vi "Main.vi"() -> ()   [LabVIEW 2023]
panel:
  in  "User interface":T1(tab)
  in  "User entries":enum32{""}(tab)
  in  "Customization":enum32{"Customization"}(tab)
  in  "Marker shape":string
  in  "Marker size":i32
  in  "PNG file path":path=path "/Users/leogallacio/Downloads/N8.png"
  in  "Colors":enum32{"Colors"}(tab)
  out "Corners":u32(colorbox)
  out "Traces":u32[](array[colorbox])
  in  "Size":enum32{"Size"}(tab)
  out "Depth":i32
  out "Width":i16
  out "Height":i16
  out "stdout":string
  out "PNG picture":picture
  out "Traces.txt":string
  out "Script.m":string
  in  "Loop FOR 1":enum32{"Loop FOR 1"}(tab)
  in  "Arrays":enum32{"Arrays"}(tab)
  out "Pixels colors (uchar)":u32[](array[numeric])
  out "Pixels colors (CLUT)":u8[](array[numeric])
  out "Corners color (CLUT)":i32
  out "Traces colors (RGB)":u8[][](array[numeric])
  out "Traces colors (CLUT)":i32[](array[numeric])
  out "Traces colors string (RGB)":string[](array[string])
  in  "Script.m":enum32{"Script.m"}(tab)
  in  "Extract.c output string scan":enum32{"Extract.c output string scan"}(tab)
  in  "T: tt1 tt2 tt3 ...":enum32{"T: tt1 tt2 tt3 ..."}(tab)
  in  "C: cc":enum32{"C: cc"}(tab)
  in  "Loop FOR 2":enum32{"Loop FOR 2"}(tab)
  out "Number of Traces":i32
  in  "LabVIEW":enum32{"LabVIEW"}(tab)
  out "VI folder":path
  out "PNG file name":string
  in  "MATLAB":enum32{"MATLAB"}(tab)
  out "Extract path":path
  out "Script.m path":path
  out "PDF file path":path
  in  "C":enum32{"C"}(tab)
  out "Pixmap.bin path":path
  out "Traces.txt path":path
  in  "MATLAB":enum32{"MATLAB"}(tab)
  out "CallMATLAB out":errorcluster
  out "CallMATLAB error":string
  in  "C":enum32{"C"}(tab)
  out "Extract.c error":string
  out "error out":errorcluster
  out "Pixmap.bin error out":errorcluster
  out "Extract error":errorcluster
  out "TracesRead error":errorcluster
  out "ScriptWrite error out":errorcluster
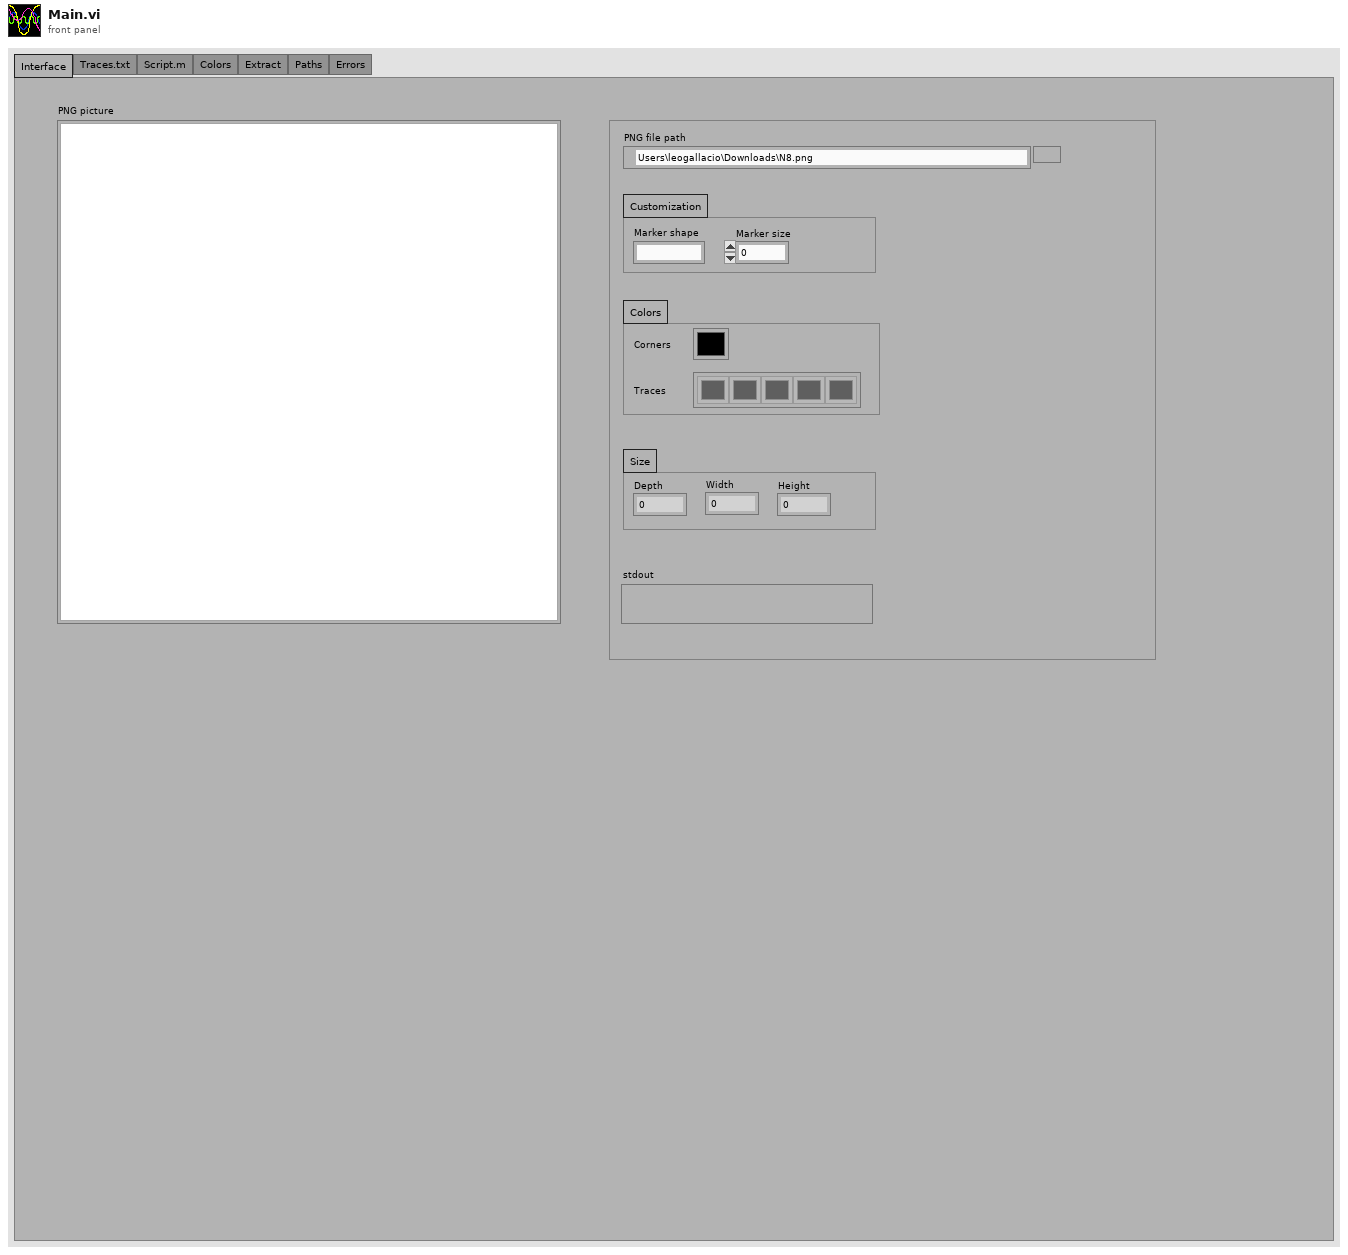
[diagram p1: front panel]
types:
  T1 = enum32{"Interface", "Traces.txt", "Script.m", "Colors", "Extract", "Paths", "Errors"}
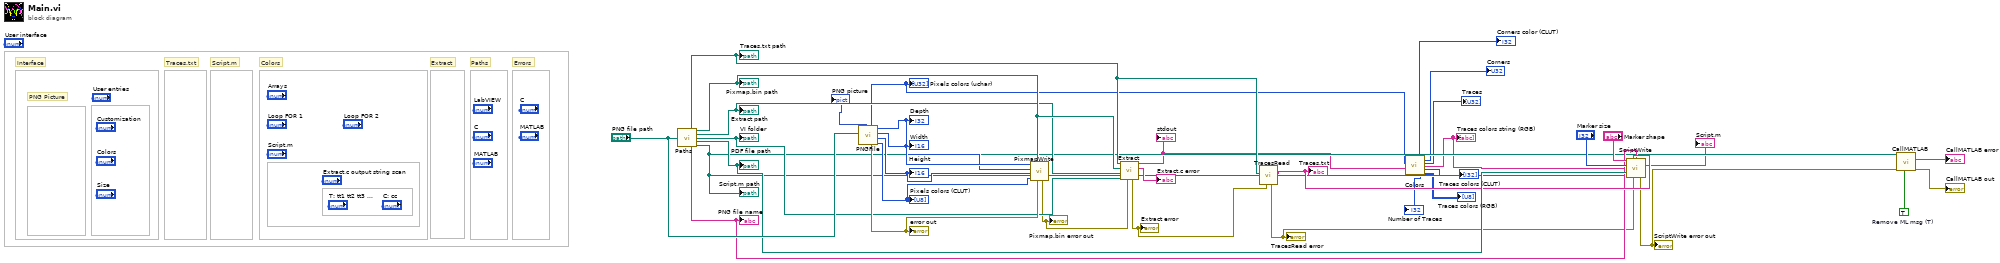
[diagram p0: block diagram]
diagram:
  w33 = TRUE  # Remove ML msg (T)
  # "PNG Picture"
  # "Errors"
  # "Paths"
  # "Extract"
  # "Colors"
  # "Script.m"
  # "Traces.txt"
  # "Interface"
  n1 = call "Paths.vi"("PNG file path"="PNG file path") -> ("Traces.txt path"=w21:path, "Pixmap.bin path"=w26:path, "Extract path"=w25:path, "VI folder"=w24:path, "PDF file path"=w17:path, "PNG file name"=w15:string, "Script.m path"=w13:path)  [unwired: 8 in]
  "Traces.txt path" <- w21
  "Pixmap.bin path" <- w26
  "Extract path" <- w25
  "VI folder" <- w24
  "PDF file path" <- w17
  "Script.m path" <- w13
  "PNG file name" <- w15
  n2 = call "PNGFile.vi"("PNG file path"="PNG file path") -> ("Pixels colors (CLUT)"=w28:u8[], "Height"=w29:i16, "Width"=w30:i16, "Depth"=w31:i32, "PNGFile error"=w27:errorcluster, "Pixels colors (uchar)"=w12:u32[], "PNG picture"=→"PNG picture":picture)  [unwired: 4 in]
  "Pixels colors (uchar)" <- w12
  "Depth" <- w31
  "Width" <- w30
  "Height" <- w29
  "Pixels colors (CLUT)" <- w28
  "error out" <- w27
  n3 = call "PixmapWrite.vi"("PNGFile error in"=w27, "Pixmap.bin path"=w26, "Pixels colors (CLUT)"=w28, "Height"=w29, "Width"=w30, "Depth"=w31) -> ("Pixmap.bin error out"=w23:errorcluster)  [unwired: 5 in]
  "Pixmap.bin error out" <- w23
  n4 = call "Extract.vi"("TracesWrite error"=w23, "VI folder"=w24, "Extract path"=w25, "Pixmap.bin path"=w26, "Traces.txt path"=w21) -> ("Extract.c error"=→"Extract.c error":string, "stdout"=w11:string, "Extract error"=w20:errorcluster)  [unwired: 4 in]
  "Extract error" <- w20
  "stdout" <- w11
  n5 = call "TracesRead.vi"("Extract error"=w20, "Traces.txt path"=w21) -> ("Traces.txt"=w16:string, "TracesRead error"=w1:errorcluster)  [unwired: 8 in]
  "TracesRead error" <- w1
  "Traces.txt" <- w16
  n6 = call "Colors.vi"("Pixels colors (uchar)"=w12, "stdout"=w11) -> ("Number of Traces"=→"Number of Traces":i32, "Corners color (CLUT)"=→"Corners color (CLUT)":i32, "Corners"=→"Corners":u32, "Traces"=→"Traces":u32[], "Traces colors string (RGB)"=w7:string[], "Traces colors (CLUT)"=→"Traces colors (CLUT)":i32[], "Traces colors (RGB)"=→"Traces colors (RGB)":u8[][])  [unwired: 11 in]
  "Traces colors string (RGB)" <- w7
  n7 = call "ScriptWrite.vi"("Marker shape"="Marker shape", "Traces.txt"=w16, "PNG file name"=w15, "Marker size"="Marker size", "Traces colors string (RGB)"=w7, "PDF file path"=w17, "Script.m path"=w13, "TracesRead error"=w1) -> ("Script.m"=→"Script.m":string, "ScriptWrite error out"=w14:errorcluster)  [unwired: 6 in]
  "ScriptWrite error out" <- w14
  n8 = call "CallMATLAB.vi"("Remove ML msg (T)"=w33, "error in (no error)"=w14, "matlab script path"=w13) -> ("error out"=→"CallMATLAB out":errorcluster, "standard error"=→"CallMATLAB error":string)  [unwired: 3 in, 4 out]
